vi "create_control.vi"(9 "Create Constant":bool, 10 "terminal index":i32, 11 "object id":string) -> (0 "error out":errorcluster, 3 "new id":string)   [LabVIEW 2026]
doc: "Creates a Control, Indicator or Constant on an objects (GObject/Node) in- or output terminal. Use get_object_terminals to get the index of the terminals. Set Create Constant to true to create a constant. Otherwise will create control/indicator based on if the terminal is input or output. Returns a reference to the newly created object."
uses:
  G-AI Core.lvlib
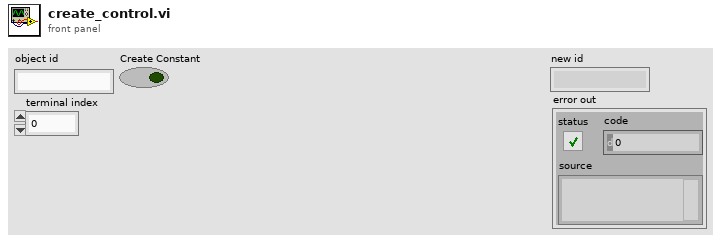
[diagram p1: front panel]
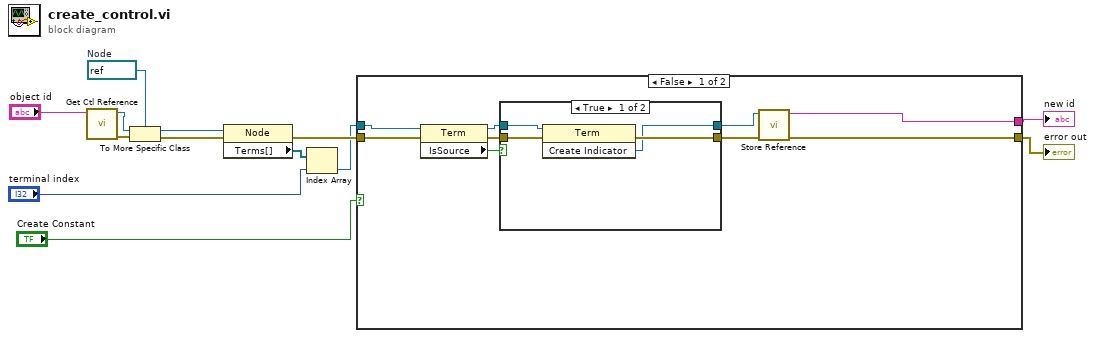
[diagram p0: block diagram]
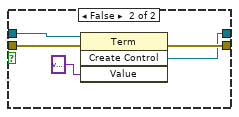
[diagram p2: hidden frame]
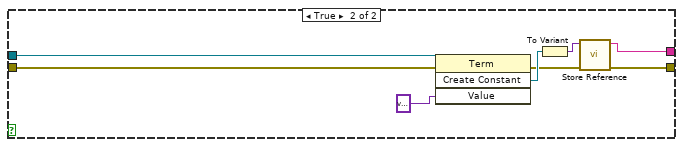
[diagram p3: hidden frame]
diagram:
  w10 = refnum<vi> refnum  # Node
  n1 = call "Get Ctl Reference.vi"("id"="object id") -> ("error out"=w12:errorcluster, "ctl reference"=w11:refnum<vi>)  [unwired: 9 in]
  n2 = To More Specific Class(target class=w10, reference=w11, error in=w12) -> (specific class reference=w7:refnum<vi>, error out=w9:errorcluster)
  n3 = property class="Node"(reference=w7, error in=w9) -> (error out=w8:errorcluster, "Terms[]"=w6:refnum<vi>[])  [unwired: 1 out]
  n4 = Index Array(array=w6, index="terminal index") -> (element=w5:refnum<vi>)
  n5 = case shown="False" "Create Constant" {
    tunnel: w8 -> [w22 w35]
    tunnel: [w16 w36] -> w1
    tunnel: w5 -> [w20 w34]
    tunnel: [w14 w33] -> w2
    frame False {
      n6 = property class="Term"(reference=w20, error in=w22) -> (reference out=w19:refnum<vi>, error out=w21:errorcluster, "IsSource"=w18:bool)
      n7 = case shown="True" w18 {
        tunnel: [w26 w31] -> w17
        tunnel: w21 -> [w25 w30]
        tunnel: w19 -> [w24 w29]
        tunnel: [w23 w28] -> w15
        frame True {
          n8 = invoke class="Term" method="Create Indicator"(reference=w24, error in=w25) -> (error out=w26:errorcluster, "Create Indicator"=w23:refnum<vi>)  [unwired: 1 in, 1 out]
        }
        frame False {
          n9 = invoke class="Term" method="Create Control"(reference=w29, error in=w30, "Value"=variant) -> (error out=w31:errorcluster, "Create Control"=w28:refnum<vi>)  [unwired: 1 in, 2 out]
        }
      }
      n10 = call "Store Reference.vi"("error in"=w17, "Reference"=w15) -> ("error out"=w16:errorcluster, "id"=w14:string)  [unwired: 8 in]
    }
    frame True {
      n11 = invoke class="Term" method="Create Constant"(reference=w34, error in=w35, "Value"=variant) -> (error out=w37:errorcluster, "Create Constant"=w39:refnum<vi>)  [unwired: 1 in, 2 out]
      n12 = To Variant(anything=w39) -> (Variant=w38:variant)
      n13 = call "Store Reference.vi"("error in"=w37, "Reference"=w38) -> ("error out"=w36:errorcluster, "id"=w33:string)  [unwired: 8 in]
    }
  }
  "new id" <- w2
  "error out" <- w1
